vi "Info Insert Row to 1D TimeStamps Array.vi"(6 "source info data":string, 7 "key description":string, 8 "sections in":string[](array[string]), 9 "row index to insert":i32, 10 "timestamp to insert":timestamp, 11 "info data in":string) -> (0 "sections out":string[](array[string]), 3 "info data out":string)   [LabVIEW 2013]
doc: "Addition to infolib: Gets 2D array of reals (if exits in the 'info data in'), inserts one row of reals into it in selected row, writes it back."
uses:
  infolib.lvlibp/Private/Get matrix polymorph parts/Get 1D Time Stamp.vi
  infolib.lvlibp/Private/Add matrix polymorph parts/1D Time Stamp.vi
  infolib.lvlibp
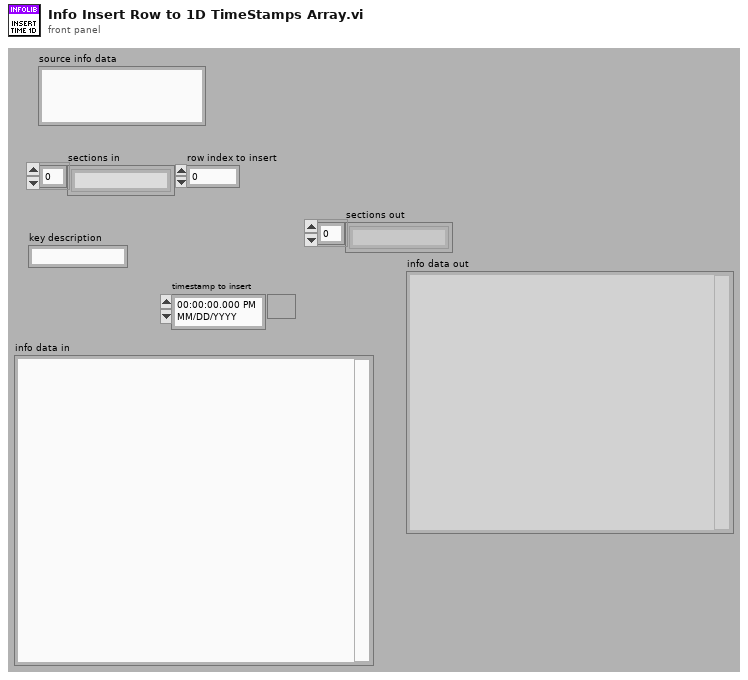
[diagram p1: front panel]
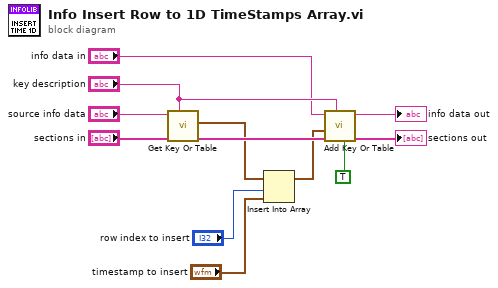
[diagram p0: block diagram]
diagram:
  n1 = call-poly "Get Key Or Table.vi"("key description"="key description", "sections"="sections in", "info data"="source info data") -> ("sections out"=w11:string[], "value"=w2:timestamp[])  [unwired: 5 in, 2 out]
  n2 = Insert Into Array(array=w2, index="row index to insert", new element="timestamp to insert") -> (w9:timestamp[])
  n3 = call-poly "Add Key Or Table.vi"("column vector (F)"=TRUE, "key description"="key description", "sections"=w11, "time stamp"=w9, "info data"="info data in") -> ("sections out"=→"sections out":string[], "info data out"=→"info data out":string)  [unwired: 5 in]
